vi "image_message_to_openai_message.vi"(8 "error in (no error)":errorcluster, 11 "message":T1) -> (0 "error out":errorcluster, 3 "OpenAI message":string)   [LabVIEW 2020, in "llm_openai_chatmodels.lvclass"]
uses:
  llm_openai_chatmodels.lvclass
  message_image/message.ctl
  message_image/message_image.lvclass
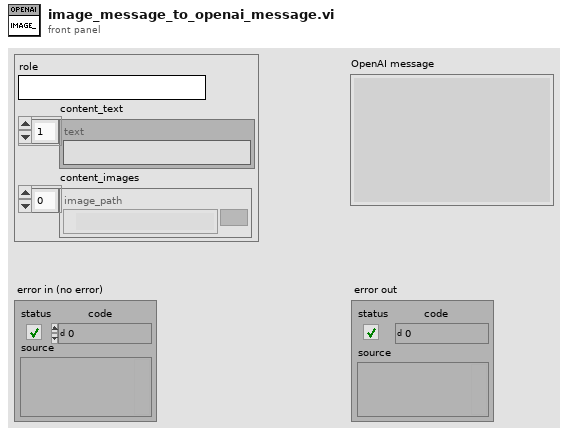
[diagram p1: front panel]
types:
  T1 = typedef "message_image.lvclass/message.ctl" = cluster{"role":string, "content_text":string[], "content_images":path[]}
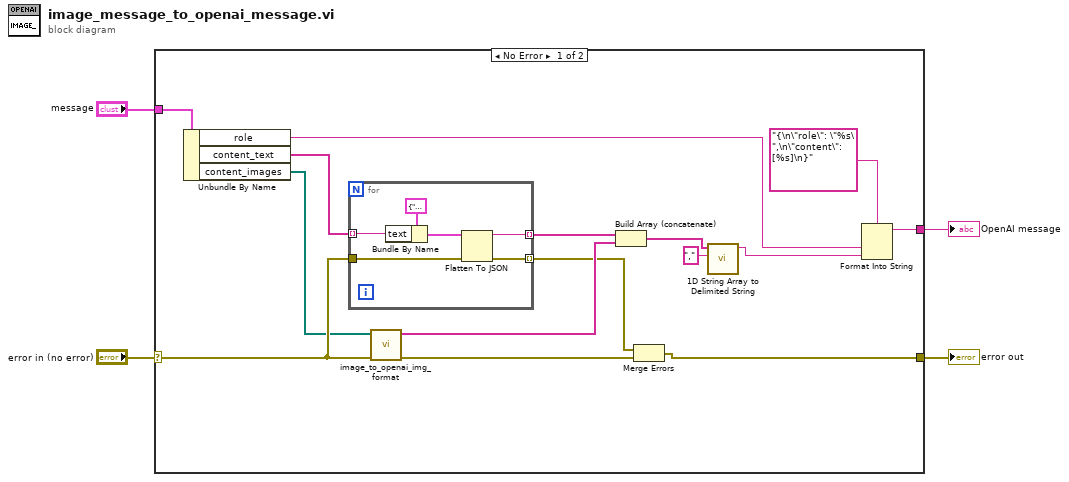
[diagram p0: block diagram]
diagram:
  n1 = case shown="No Error" "error in (no error)" {
    selector: "error in (no error)" -> [w11 w26]
    tunnel: "message" -> [w19 _]
    tunnel: [w14 _] -> w2
    tunnel: [w5 w26] -> w1
    frame No Error {
      n2 = Unbundle By Name(w19) -> ("role"=w15:string, "content_text"=w13:string[], "content_images"=w10:path[])
      n3 = for {
        tunnel: w13 -> [w25] mode=indexing
        tunnel: [w20] -> w12 mode=indexing
        tunnel: w11 -> [w22]
        tunnel: [w21] -> w6 mode=indexing
        n4 = Bundle By Name(cluster=cluster{"type":string, "text":string} {"type"="text", "text"=""} ("parts"), "text"=w25) -> (w23:cluster{"type":string, "text":string})
        n5 = Flatten To JSON(anything=w23, error in (no error)=w22) -> (JSON string=w20:string, 11:w21:errorcluster)  [unwired: 1 in]
      }
      n6 = call "image_to_openai_img_format.vi"("error in (no error)"=w11, "imagepaths"=w10) -> ("error out"=w7:errorcluster, "image_data"=w8:string[])  [unwired: 8 in]
      n7 = Build Array (concatenate)(w12, w8) -> (w9:string[])
      n8 = Merge Errors(w6, w7) -> (w5:errorcluster)
      n9 = call <vilib>:"1D String Array to Delimited String.vi"("delimiter"=",", "string array"=w9) -> ("delimited string"=w16:string)  [unwired: 9 in]
      n10 = Format Into String(format string="{\n\"role\": \"%s\",\n\"content\": [%s]\n}", w15, w16) -> (resulting string=w14:string)  [unwired: 2 in, 1 out]
    }
    frame Error {
    }
  }
  "error out" <- w1
  "OpenAI message" <- w2
